vi "plot_parseYoung.vi"(0 "Current Data":dbl[][](array[numeric]), 5 "Yesterday's Data":dbl[][](array[numeric])) -> (4 "Plot 1":T1(array[cluster]), 8 "Plot 2":T2(array[cluster]), 15 "Plot 3":T3(array[cluster]))   [LabVIEW 2018]
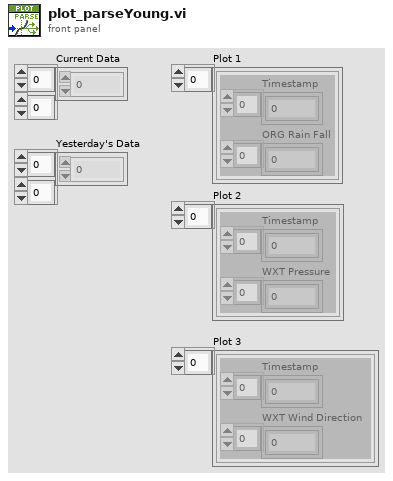
[diagram p1: front panel]
types:
  T1 = cluster{"Timestamp":dbl[], "ORG Rain Fall":dbl[]}[]
  T2 = cluster{"Timestamp":dbl[], "WXT Pressure":dbl[]}[]
  T3 = cluster{"Timestamp":dbl[], "WXT Wind Direction":dbl[]}[]
  T4 = cluster{"Timestamp":dbl[], "Young Temperature":dbl[], "Young Rain Rate":dbl[], "Young Rain Fall":dbl[], "Young Humidity":dbl[], "Young Pressure":dbl[], "Young Wind Speed":dbl[], "Young Wind Direction":dbl[]}
  T5 = cluster{"Timestamp":dbl[], "Young Temperature":dbl[]}
  T6 = cluster{"Timestamp":dbl[], "Young Rain Fall":dbl[]}
  T7 = cluster{"Timestamp":dbl[], "Young Humidity":dbl[]}
  T8 = cluster{"Timestamp":dbl[], "Young Pressure":dbl[]}
  T9 = cluster{"Timestamp":dbl[], "Young Wind Speed":dbl[]}
  T10 = cluster{"Timestamp":dbl[], "Young Wind Direction":dbl[]}
  T11 = cluster{"Timestamp":dbl[], "Young Rain Fall":dbl[]}[]
  T12 = cluster{"Timestamp":dbl[], "Young Pressure":dbl[]}[]
  T13 = cluster{"Timestamp":dbl[], "Young Wind Direction":dbl[]}[]
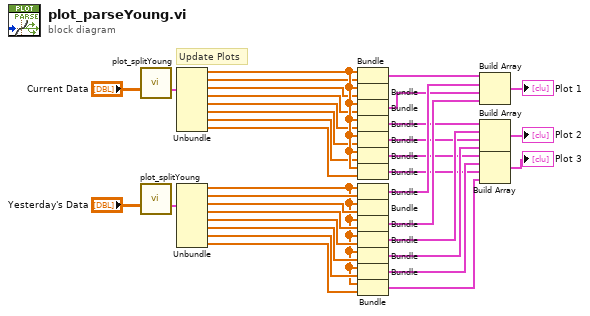
[diagram p0: block diagram]
diagram:
  # "Update Plots"
  n1 = call "plot_splitYoung.vi"("Input Arrays"="Current Data") -> ("output cluster"=w13:T4)  [unwired: 14 in]
  n2 = call "plot_splitYoung.vi"("Input Arrays"="Yesterday's Data") -> ("output cluster"=w30:T4)  [unwired: 14 in]
  n3 = Unbundle(w13) -> ("Timestamp"=w21:dbl[], "Young Temperature"=w14:dbl[], "Young Rain Rate"=w15:dbl[], "Young Rain Fall"=w16:dbl[], "Young Humidity"=w17:dbl[], "Young Pressure"=w18:dbl[], "Young Wind Speed"=w19:dbl[], "Young Wind Direction"=w20:dbl[])
  n4 = Unbundle(w30) -> ("Timestamp"=w22:dbl[], "Young Temperature"=w29:dbl[], "Young Rain Rate"=w28:dbl[], "Young Rain Fall"=w27:dbl[], "Young Humidity"=w26:dbl[], "Young Pressure"=w25:dbl[], "Young Wind Speed"=w24:dbl[], "Young Wind Direction"=w23:dbl[])
  n5 = Bundle("Timestamp"=w21, "Young Temperature"=w14) -> (w31:T5)  [unwired: 1 in]
  n6 = Bundle("Timestamp"=w21, "Young Rain Rate"=w15) -> ()  [unwired: 1 in, 1 out]
  n7 = Bundle("Timestamp"=w21, "Young Rain Fall"=w16) -> (w12:T6)  [unwired: 1 in]
  n8 = Bundle("Timestamp"=w21, "Young Humidity"=w17) -> (w10:T7)  [unwired: 1 in]
  n9 = Bundle("Timestamp"=w21, "Young Pressure"=w18) -> (w8:T8)  [unwired: 1 in]
  n10 = Bundle("Timestamp"=w21, "Young Wind Speed"=w19) -> (w5:T9)  [unwired: 1 in]
  n11 = Bundle("Timestamp"=w21, "Young Wind Direction"=w20) -> (w2:T10)  [unwired: 1 in]
  n12 = Bundle("Timestamp"=w22, "Young Temperature"=w29) -> (w32:T5)  [unwired: 1 in]
  n13 = Bundle("Timestamp"=w22, "Young Rain Rate"=w28) -> ()  [unwired: 1 in, 1 out]
  n14 = Bundle("Timestamp"=w22, "Young Rain Fall"=w27) -> (w11:T6)  [unwired: 1 in]
  n15 = Bundle("Timestamp"=w22, "Young Humidity"=w26) -> (w9:T7)  [unwired: 1 in]
  n16 = Bundle("Timestamp"=w22, "Young Pressure"=w25) -> (w7:T8)  [unwired: 1 in]
  n17 = Bundle("Timestamp"=w22, "Young Wind Speed"=w24) -> (w4:T9)  [unwired: 1 in]
  n18 = Bundle("Timestamp"=w22, "Young Wind Direction"=w23) -> (w1:T10)  [unwired: 1 in]
  n19 = Build Array(w31, w32, w12, w11) -> (→"Plot 1":T11)
  n20 = Build Array(w10, w9, w8, w7) -> (→"Plot 2":T12)
  n21 = Build Array(w5, w4, w2, w1) -> (→"Plot 3":T13)
